vi "Write Prefix.vi"(8 "error in (no error)":errorcluster, 10 "Prefix":string, 11 "Lakeshore 331 in":refnum<class "Lakeshore 331.lvclass">) -> (0 "error out":errorcluster, 3 "Lakeshore 331 out":refnum<class "Lakeshore 331.lvclass">)   [LabVIEW 2022 SP3, in "Lakeshore 331.lvclass"]
uses:
  Lakeshore 331.lvclass
  Lakeshore 331.lvclass/Lakeshore 331.ctl
  Temp Control.lvclass
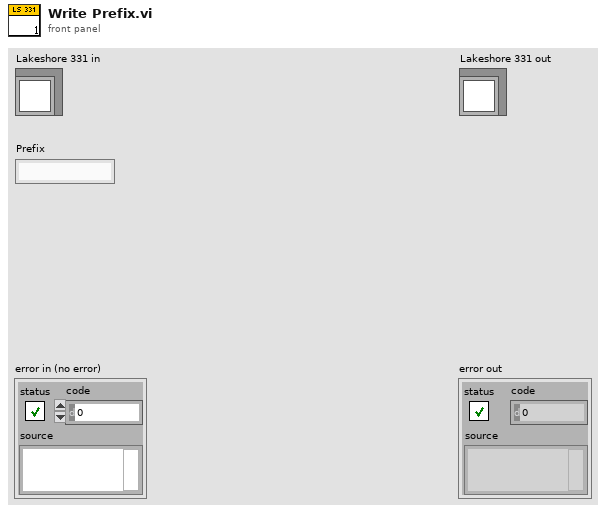
[diagram p1: front panel]
types:
  T1 = typedef "Lakeshore 331.lvclass/Lakeshore 331 Settings.ctl" = cluster{"Addr":refnum<visa-resource-name>, "Ch Prefix":string, "Ch Select":i32[]}
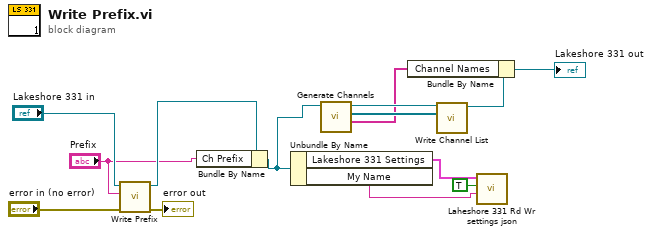
[diagram p0: block diagram]
diagram:
  n1 = call-parent "Write Prefix.vi"("error in (no error)"="error in (no error)", "Prefix"="Prefix", "Temp Control in"="Lakeshore 331 in") -> ("error out"=→"error out":errorcluster, "Temp Control out"=w11:refnum<class "Lakeshore 331.lvclass">)  [unwired: 7 in]
  n2 = Bundle By Name(cluster=w11, "Ch Prefix"="Prefix") -> (w6:refnum<class "Lakeshore 331.lvclass">)
  n3 = Unbundle By Name(w6) -> ("Lakeshore 331 Settings"=w9:T1, "My Name"=w7:string)
  n4 = call-dynamic "Generate Channels.vi"("Lakeshore 331 in"=w6) -> ("Channel Names"=w3:string[], "Channel List"=w5:refnum<class "HK Item.lvclass">[], "Lakeshore 331 out"=w4:refnum<class "Lakeshore 331.lvclass">)  [unwired: 7 in, 1 out]
  n5 = call-dynamic "Write Channel List.vi"("Channel List"=w5, "Temp Control in"=w4) -> ("Temp Control out"=w1:refnum<class "Lakeshore 331.lvclass">)  [unwired: 8 in, 1 out]
  n6 = Bundle By Name(cluster=w1, "Channel Names"=w3) -> (→"Lakeshore 331 out":refnum<class "Lakeshore 331.lvclass">)
  n7 = call "Laheshore 331 Rd Wr settings json.vi"("section"=w7, "Write? (F:Read)"=TRUE, "Lakeshore 331 Settings"=w9) -> ()  [unwired: 7 in, 2 out]
